vi "Numeric Indicator - Integer.vi"() -> ()   [LabVIEW 2012]
doc: "Sample numeric display item."
uses:
  <vilib>/NI Veristand/Display Template Support/Display Template Support.llb/cluster_Screen Item Settings.ctl
  <vilib>/NI Veristand/Display Template Support/Display Template Support.llb/cluster_Graph Scale Settings.ctl
  <vilib>/NI Veristand/Display Template Support/Display Template Support.llb/cluster_Graph Plot Settings.ctl
  NationalInstruments.VeriStand.SystemStorage
  <vilib>/NI Veristand/Display Template Support/Display Template Support.llb/enum_Display Template Handler Minimal To Widget Msg.ctl
  <vilib>/NI Veristand/Display Template Support/Display Template Support.llb/enum_Display Template Handler Minimal To Workspace.ctl
  Integer Object Parameters.ctl
  <vilib>/NI Veristand/Execution/Workspace/NI_VS Workspace ExecutionAPI.lvlib
panel:
  in  "NIVS.System Definition Root":refnum<k24>
  in  "NIVS.Gateway IP Address":string
  out "Numeric":i64
  out "Label":string="Numeric"
  in  "Item.Data":T1
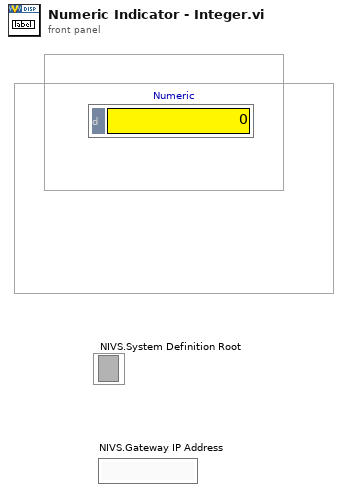
[diagram p1: front panel]
types:
  T1 = typedef "cluster_Screen Item Settings.ctl" = cluster{"Template VI":string, "Position X":i32, "Position Y":i32, "Custom":string, "Show Title Bar":bool, "ID":i32, "Always On Top":bool, "Allow Resize":bool, "Allow Minimize":bool, "Allow Close":bool, "Size to Screen":bool, "Screen.ID":i32, "State":enum16{"Normal", "New"}, "Title":string, "Window Bounds":cluster{"[0]":i16, "[1]":i16, "[2]":i16, "[3]":i16}, "Channel Ref":u64, "Unit":string, "Default Units?":bool, "Flash Limit?":bool, "Color 1":u32, "Color 2":u32, "Color 3":u32, "Color 4":u32, "Bck Color":u32, "Fore Color":u32, "Limit 1":dbl, "Limit 2":dbl, "Limit 3":dbl, "Limit 4":dbl, "Limit Mode 1":i32, "Limit Mode 2":i32, "Limit Mode 3":i32, "Limit Mode 4":i32, "Scale Precision":i32, "Scale Min":dbl, "Scale Max":dbl, "Format":i32, "Precision":i32, "Background Type":i32, "IDs":i32[], "Units":string[], "Labels":string[], "Scale Factor":dbl, "Scale Offset":dbl, "YScale Index":u32[], "XScale":T2, "YScales":T2[], "Plots":T3[], "Update Period":dbl, "History Length":dbl, "My.Ref":refnum<vi>, "Is Control?":bool, "Channel Paths":string[], "Custom Data":variant}
  T2 = typedef "cluster_Graph Scale Settings.ctl" = cluster{"Format":u8, "Precision":u8, "Fit":u8, "Label":string, "Use Default Label":bool, "Label Visible":bool, "Min":dbl, "Max":dbl}
  T3 = typedef "cluster_Graph Plot Settings.ctl" = cluster{"Bar Style":u8, "Fill To":i16, "Fill/PtColor":u32, "Line Style":u8, "Line Width":u8, "Color":u32, "Interp":u8, "Point Style":u8}
  T4 = typedef "enum_Display Template Handler Minimal To Workspace.ctl" = cluster{"Operation":enum16{"SetCustomData", "DeleteItem"}, "Data":variant}
  T5 = typedef "enum_Display Template Handler Minimal To Widget Msg.ctl" = enum16{"Stop", "LaunchConfigDialog"}
  T6 = typedef "Integer Object Parameters.ctl" = cluster{"Node Path":string, "NodePathArray":string[], "Integer":cluster{"Label":string, "Digits of Precision":u8, "Integer Format":enum8{"Decimal", "Scientific", "Engineering", "Binary", "Octal", "Hexadecimal", "Relative Time", "Time and Date", "SI"}}}
  T7 = enum8{"Decimal", "Scientific", "Engineering", "Binary", "Octal", "Hexadecimal", "Relative Time", "Time and Date", "SI"}
  T8 = typedef "NI_VS Workspace ExecutionAPI.lvlib/WorkspaceAPI.ctl" = refnum<k24>
  T9 = cluster{"Node Path":string, "NodePathArray":string[], "Integer":cluster{"Label":string, "Digits of Precision":u8, "Integer Format":enum8{"Decimal", "Scientific", "Engineering", "Binary", "Octal", "Hexadecimal", "Relative Time", "Time and Date", "SI"}}}
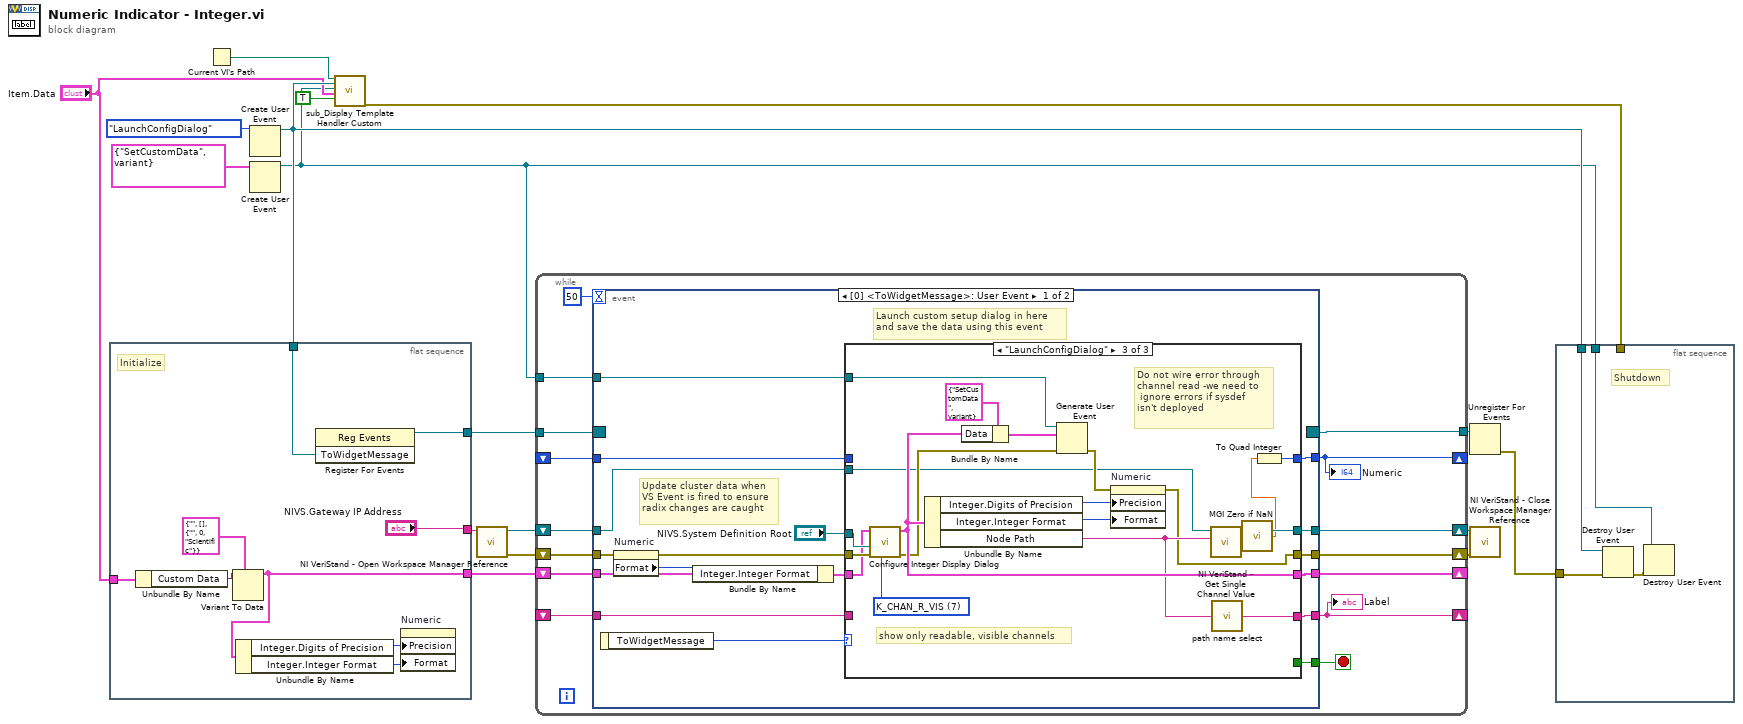
[diagram p0: block diagram]
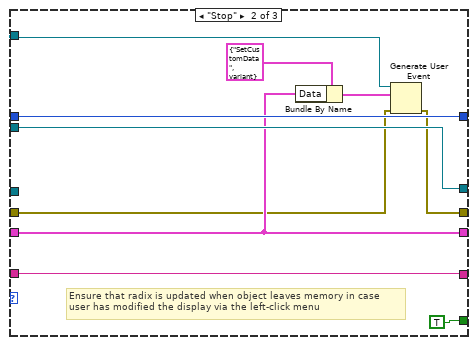
[diagram p3: hidden frame]
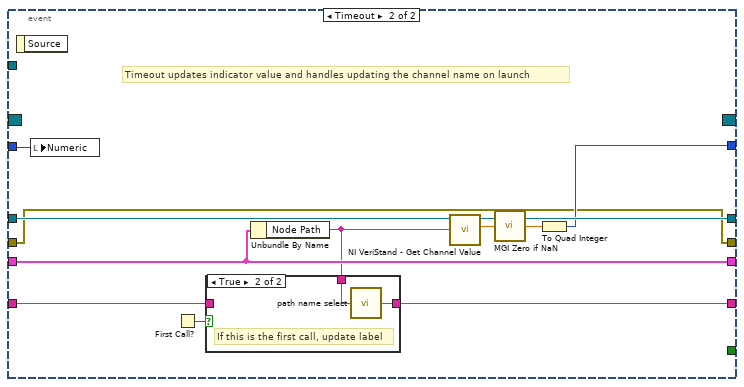
[diagram p4: hidden frame]
diagram:
  n1 = flat-sequence {
    tunnel: [w26] -> w15
    tunnel: w12 -> [w25]
    tunnel: "Item.Data" -> [w24]
    tunnel: [w20] -> w6
    tunnel: ["NIVS.Gateway IP Address"] -> w1
    frame #0 {
      # "Initialize"
      n2 = Unbundle By Name(w24) -> ("Custom Data"=w23:variant)
      n3 = Variant To Data(type=T6 {"Node Path"="", "NodePathArray"=[], "Integer"={"Label"="", "Digits of Precision"=0, "Integer Format"=enum."Scientific"}}, Variant=w23) -> (data=w20:T6)  [unwired: 1 in, 1 out]
      n4 = Unbundle By Name(w20) -> ("Integer.Digits of Precision"=w19:u8, "Integer.Integer Format"=w18:T7)
      n5 = register-events(w25) -> (reference out=w26:refnum<event-registration>)  [unwired: 2 in, 1 out]
      n6 = property on="Numeric" class="DigNum (strict)"("Precision"=w19, "Format"=w18) -> ()  [unwired: 2 in, 2 out]
    }
  }
  n7 = Current VI's Path() -> (path=w10:path)
  n8 = Create User Event(user event datatype=enum_Display_Template_Handler_Minimal_To_Widget_Msg."LaunchConfigDialog" ("ToWidgetMessage")) -> (user event=w12:refnum<user-event>)  [unwired: 1 in, 1 out]
  n9 = Create User Event(user event datatype=T4 {"Operation"=enum."SetCustomData", "Data"=variant} ("Data")) -> (user event=w8:refnum<user-event>)  [unwired: 1 in, 1 out]
  n10 = call <vilib>:"sub_Display Template Handler Custom.vi"("Parent.Path"=w10, "ToWidgetEvent"=w12, "ToWorkspace"=w8, "Item.Data"="Item.Data", "Resizable"=TRUE) -> ("error out"=w17:errorcluster)  [unwired: 14 in]
  n11 = call <vilib>:"NI VeriStand - Open Workspace Manager Reference.vi"("Gateway IP Address (\"\": localhost)"=w1) -> ("error out"=w4:errorcluster, "WorkspaceManager"=w5:T8)  [unwired: 9 in]
  n12 = while {
    tunnel: w15 -> [w41]
    tunnel: [w39] -> w14
    tunnel: w8 -> [w38]
    shift-right: [w30] -> _
    shift-left: w6 -> [w37]
    shift-right: [w33] -> w3
    shift-left: w5 -> [w35]
    shift-right: [w32] -> w2
    shift-left: w4 -> [w34]
    shift-right: [w27] -> _
    shift-left: _ -> [w31]
    shift-right: [w28] -> _
    shift-left: _ -> [w29]
    stop <- w40 stop-if-true
    n13 = event shown="[0] <ToWidgetMessage>: User Event" {
      selector: w41 -> [_ _]
      dyn-events: [_ _] -> w39
      timeout: 50 -> [_ _]
      tunnel: [w57 _] -> w40
      tunnel: w38 -> [w56 _]
      tunnel: [w55 w101] -> w30
      tunnel: w37 -> [w42 w101]
      tunnel: [w54 w99] -> w27
      tunnel: w35 -> [w53 w102]
      tunnel: w34 -> [w44 w94]
      tunnel: [w52 w100] -> w33
      tunnel: [w51 w94] -> w32
      tunnel: w31 -> [w50 w98]
      tunnel: [w48 w103] -> w28
      tunnel: w29 -> [w47 w104]
      event User Event {
        # "Update cluster data when\nVS Event is fired to ensure\nradix changes are caught"
        # "Launch custom setup dialog in here\nand save the data using this event"
        n14 = event-data() -> ("ToWidgetMessage"=w58:T5)  [unwired: 1 out]
        n15 = property on="Numeric" class="DigNum (strict)"(error in=w44) -> (error out=w45:errorcluster, "Format"=w46:u8)  [unwired: 1 in, 1 out]
        n16 = Bundle By Name(cluster=w42, "Integer.Integer Format"=w46) -> (w43:T6)
        n17 = case shown="\"LaunchConfigDialog\"" w58 {
          tunnel: [_ TRUE _] -> w57
          tunnel: w56 -> [_ w67 w93]
          tunnel: [w63 w65 w87] -> w55
          tunnel: w43 -> [w63 w65 w88]
          tunnel: [w60 w71 w78] -> w54
          tunnel: w53 -> [w62 w72 w81]
          tunnel: w45 -> [w61 w64 w90]
          tunnel: [w62 w72 w79] -> w52
          tunnel: [w61 w66 w74] -> w51
          tunnel: w50 -> [w60 w71 _]
          tunnel: "NIVS.System Definition Root" -> [_ _ w89]
          tunnel: [w59 w70 w82] -> w48
          tunnel: w47 -> [w59 w70 _]
          frame Default {
          }
          frame "Stop" {
            # "Ensure that radix is updated when object leaves memory in case\nuser has modified the display via the left-click menu"
            n18 = Bundle By Name(cluster=T4 {"Operation"=enum."SetCustomData", "Data"=variant} ("event data"), "Data"=w65) -> (w68:T4)
            n19 = Generate User Event(user event=w67, event data cluster=w68, error in=w64) -> (error out=w66:errorcluster)  [unwired: 1 out]
          }
          frame "LaunchConfigDialog" {
            w75 = u8 7 items=["K_CHAN_R", "K_CHAN_W", "K_CHAN_RW", "K_CHAN_VOLT", "K_CHAN_FAULT", "K_ALL", "K_CUSTOM", "K_CHAN_R_VIS", "K_CHAN_W_VIS", "K_CHAN_RW_VIS", "K_CHAN_VOLT_VIS", "K_CHAN_FAULT_VIS"] ("DisplayFilter")
            # "Do not wire error through\nchannel read -we need to\n ignore errors if sysdef \nisn't deployed"
            # "show only readable, visible channels"
            n20 = call "Configure Integer Display Dialog.vi"("DisplayFilter"=w75, "error in (no error)"=w90, "NIVS.System Definition Root"=w89, "Data cluster in"=w88) -> ("error out"=w84:errorcluster, "Data cluster out"=w87:T9)  [unwired: 6 in]
            n21 = Unbundle By Name(w87) -> ("Integer.Digits of Precision"=w86:u8, "Integer.Integer Format"=w85:T7, "Node Path"=w80:string)
            n22 = Bundle By Name(cluster=T4 {"Operation"=enum."SetCustomData", "Data"=variant} ("event data"), "Data"=w87) -> (w91:T4)
            n23 = Generate User Event(user event=w93, event data cluster=w91, error in=w84) -> (error out=w83:errorcluster)  [unwired: 1 out]
            n24 = property on="Numeric" class="DigNum (strict)"(error in=w83, "Precision"=w86, "Format"=w85) -> (error out=w74:errorcluster)  [unwired: 1 in, 1 out]
            n25 = call <vilib>:"NI VeriStand - Get Single Channel Value.vi"("Channel"=w80, "WorkspaceManager in"=w81) -> ("Value"=w77:dbl, "WorkspaceManager out"=w79:T8)  [unwired: 7 in, 1 out]
            n26 = call "path name select.vi"("In"=w80) -> ("Out"=w82:string)
            n27 = call <userlib>:"MGI Zero if NaN.vi"("Number In"=w77) -> ("Number Out"=w76:dbl)
            n28 = To Quad Integer(1:w76) -> (0:w78:i64)
          }
        }
      }
      event Timeout {
        # "Timeout updates indicator value and handles updating the channel name on launch"
        n29 = event-data() -> ()  [unwired: 2 out]
        n30 = local write "Numeric"(w98) -> ()
        n31 = First Call?() -> (First Call?: T/F=w105:bool)
        n32 = Unbundle By Name(w101) -> ("Node Path"=w97:string)
        n33 = case shown="True" w105 {
          tunnel: w104 -> [w106 _]
          tunnel: [w106 w108] -> w103
          tunnel: w97 -> [_ w107]
          frame False {
          }
          frame True {
            # "If this is the first call, update label"
            n34 = call "path name select.vi"("In"=w107) -> ("Out"=w108:string)
          }
        }
        n35 = call-poly <vilib>:"NI VeriStand - Get Channel Value.vi"("Channel"=w97, "WorkspaceManager in"=w102) -> ("Value"=w96:dbl, "WorkspaceManager out"=w100:T8)  [unwired: 7 in, 1 out]
        n36 = call <userlib>:"MGI Zero if NaN.vi"("Number In"=w96) -> ("Number Out"=w95:dbl)
        n37 = To Quad Integer(1:w95) -> (0:w99:i64)
      }
    }
    "Label" <- w28
    "Numeric" <- w27
  }
  n38 = Unregister For Events(event registration refnum=w14) -> (error out=w13:errorcluster)  [unwired: 1 in]
  n39 = call <vilib>:"NI VeriStand - Close Workspace Manager Reference.vi"("error in (no error)"=w2, "WorkspaceManager"=w3) -> ()  [unwired: 9 in, 1 out]
  n40 = flat-sequence {
    tunnel: w17 -> [_]
    tunnel: w13 -> [w111]
    tunnel: w12 -> [w112]
    tunnel: w8 -> [w109]
    frame #0 {
      # "Shutdown"
      n41 = Destroy User Event(user event=w112, error in=w111) -> (error out=w110:errorcluster)
      n42 = Destroy User Event(user event=w109, error in=w110) -> ()  [unwired: 1 out]
    }
  }
